vi "Project 1.vi"() -> ()   [LabVIEW 2023]
panel:
  out "Is Delta greater than 0?":bool
  out "X2":dbl
  out "X1":dbl
  in  "c":i8(slide) min=-10 max=10 scale=0.0..10.0
  in  "b":i8(slide) min=-10 max=10 scale=0.0..10.0
  in  "a":i8(slide) min=-10 max=10 scale=0.0..10.0
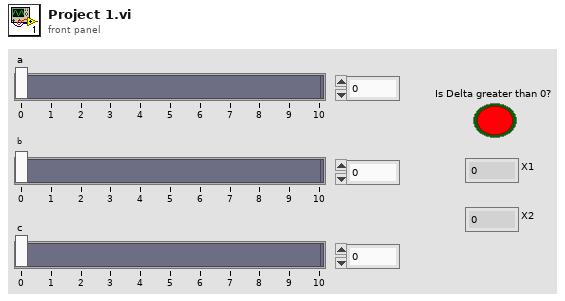
[diagram p1: front panel]
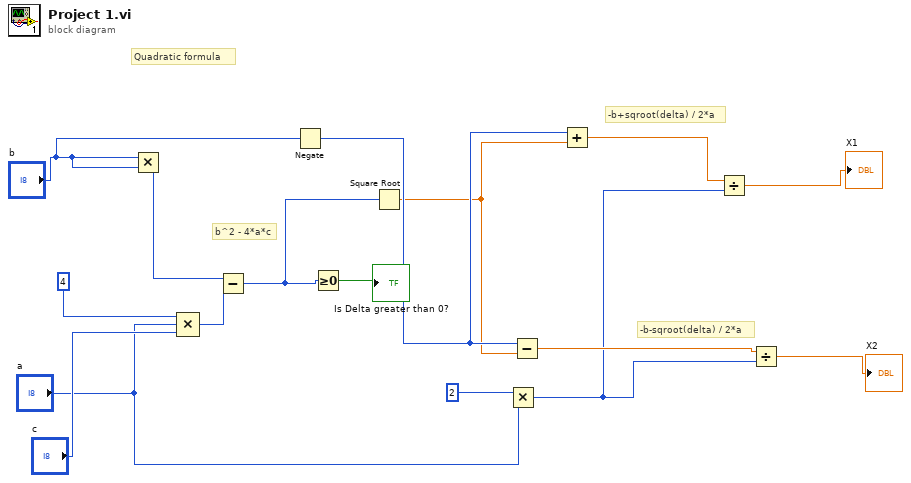
[diagram p0: block diagram]
diagram:
  # "-b-sqroot(delta) / 2*a"
  # "-b+sqroot(delta) / 2*a"
  # "b^2 - 4*a*c"
  # "Quadratic formula"
  n1 = Multiply(x="b", y="b") -> (x*y=w14:i8)
  n2 = Compound Arithmetic op=MULTIPLY(4, "a", "c") -> (w13:i32)
  n3 = Subtract(x=w14, y=w13) -> (x-y=w10:i32)
  n4 = Negate(x="b") -> (-x=w5:i8)
  n5 = Greater Or Equal To 0?(x=w10) -> (x >= 0?=→"Is Delta greater than 0?":bool)
  n6 = Square Root(x=w10) -> (sqrt(x)=w4:dbl)
  n7 = Multiply(x=2, y="a") -> (x*y=w2:i32)
  n8 = Subtract(x=w5, y=w4) -> (x-y=w6:dbl)
  n9 = Add(x=w5, y=w4) -> (x+y=w3:dbl)
  n10 = Divide(x=w3, y=w2) -> (x/y=→"X1":dbl)
  n11 = Divide(x=w6, y=w2) -> (x/y=→"X2":dbl)
